vi "Norm graph.vi"(8 "error in (no error)":errorcluster, 9 "#kinetics":i32=2 min=2 step=1, 10 "Combo Box":string(combo)="Kinetics", 11 "Control-Client in":refnum<class "Control-Client.lvclass">) -> (0 "error out":errorcluster, 3 "Control-Client out":refnum<class "Control-Client.lvclass">)   [LabVIEW 2018, in "Control-Client.lvclass"]
uses:
  Control-Client.lvclass
  Control-Client.lvclass/Control-Client.ctl
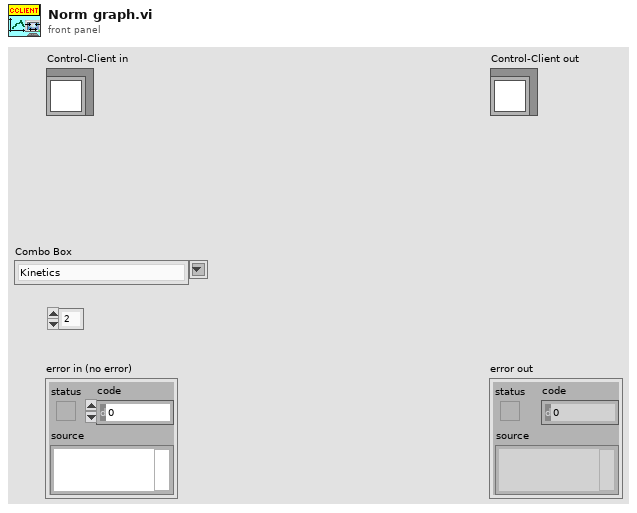
[diagram p1: front panel]
types:
  T1 = cluster{"waves slider":refnum<vi>, "times slider":refnum<vi>}
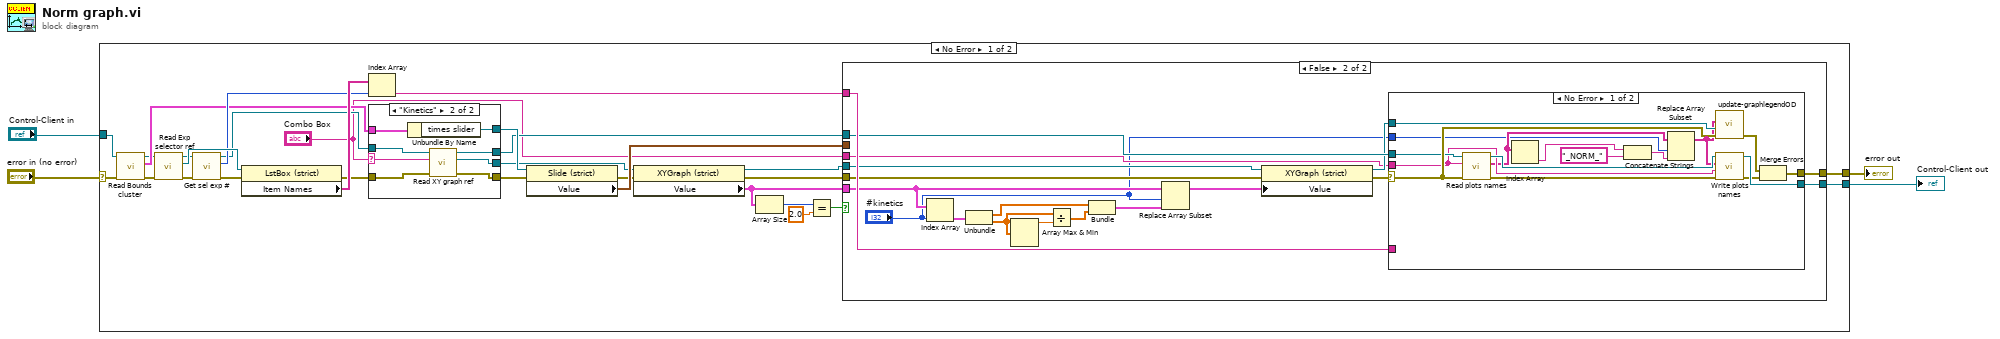
[diagram p0: block diagram]
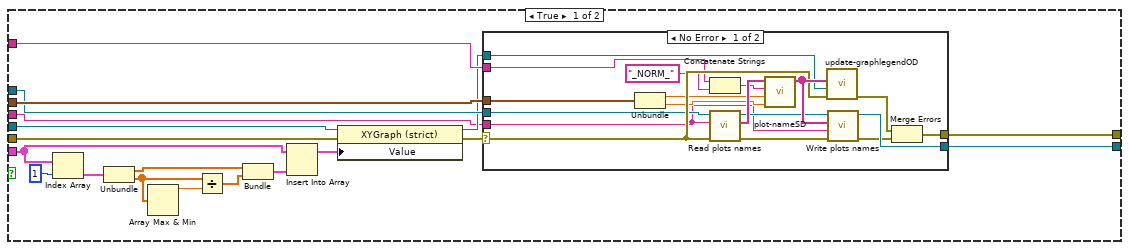
[diagram p2: hidden frame]
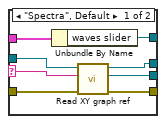
[diagram p5: hidden frame]
diagram:
  n1 = case shown="No Error" "error in (no error)" {
    selector: "error in (no error)" -> [w8 w126]
    tunnel: "Control-Client in" -> [w18 w125]
    tunnel: [w17 w126] -> w3
    tunnel: [w16 w125] -> w2
    frame No Error {
      n2 = call "Read Bounds cluster.vi"("error in (no error)"=w8, "Control-Client in"=w18) -> ("error out"=w7:errorcluster, "Bounds cluster"=w26:T1, "Control-Client out"=w9:refnum<class "Control-Client.lvclass">)  [unwired: 7 in]
      n3 = call "Read Exp selector ref.vi"("error in (no error)"=w7, "Control-Client in"=w9) -> ("error out"=w6:errorcluster, "Exp selector ref"=w30:refnum<vi>, "Control-Client out"=w10:refnum<class "Control-Client.lvclass">)  [unwired: 7 in]
      n4 = call "Get sel exp #.vi"("error in (no error)"=w6, "Control-Client in"=w10) -> ("error out"=w5:errorcluster, "Exp sel #"=w28:i32, "Control-Client out"=w24:refnum<class "Control-Client.lvclass">)  [unwired: 7 in]
      n5 = property class="LstBox (strict)"(reference=w30, error in=w5) -> (error out=w25:errorcluster, "Item Names"=w29:string[])  [unwired: 1 out]
      n6 = Index Array(array=w29, index=w28) -> (element=w31:string)
      n7 = case shown="\"Kinetics\"" "Combo Box" {
        selector: "Combo Box" -> [w116 w118]
        tunnel: [w113 w124] -> w22
        tunnel: [w112 w123] -> w27
        tunnel: w24 -> [w114 w122]
        tunnel: w25 -> [w115 w121]
        tunnel: w26 -> [w111 w120]
        tunnel: [w110 w119] -> w33
        tunnel: [w109 w117] -> w23
        frame "Spectra", Default {
          n8 = Unbundle By Name(w111) -> ("waves slider"=w110:refnum<vi>)
          n9 = call "Read XY graph ref.vi"("error in (no error)"=w115, "Combo Box"=w116, "Control-Client in"=w114) -> ("error out"=w112:errorcluster, "XY graph ref"=w113:refnum<vi>, "Control-Client out"=w109:refnum<class "Control-Client.lvclass">)  [unwired: 6 in]
        }
        frame "Kinetics" {
          n10 = Unbundle By Name(w120) -> ("times slider"=w119:refnum<vi>)
          n11 = call "Read XY graph ref.vi"("error in (no error)"=w121, "Combo Box"=w118, "Control-Client in"=w122) -> ("error out"=w123:errorcluster, "XY graph ref"=w124:refnum<vi>, "Control-Client out"=w117:refnum<class "Control-Client.lvclass">)  [unwired: 6 in]
        }
      }
      n12 = property class="Slide (strict)"(reference=w33, error in=w27) -> (error out=w20:errorcluster, "Value"=w32:cluster{dbl, dbl})  [unwired: 1 out]
      n13 = property class="XYGraph (strict)"(reference=w22, error in=w20) -> (reference out=w21:refnum<vi>, error out=w19:errorcluster, "Value"=w14:cluster{"Y":dbl[], "Y":dbl[]}[])
      n14 = Array Size(array=w14) -> (size(s)=w13:i32)
      n15 = Equal?(x=w13, y=2.0) -> (x = y?=w12:bool)
      n16 = case shown="False" w12 {
        tunnel: w32 -> [w52 _]
        tunnel: w31 -> [w51 w90]
        tunnel: w23 -> [w50 w89]
        tunnel: w21 -> [w49 w88]
        tunnel: w14 -> [w46 w77]
        tunnel: w19 -> [w44 w86]
        tunnel: [w37 w80] -> w17
        tunnel: [w36 w79] -> w16
        tunnel: "Combo Box" -> [w34 w74]
        frame True {
          n17 = Index Array(array=w46, index=1) -> (element=w42:cluster{"Y":dbl[], "Y":dbl[]})
          n18 = Unbundle(w42) -> ("Y"=w39:dbl[], "Y"=w41:dbl[])
          n19 = Array Max & Min(array=w41) -> (max value=w35:dbl)  [unwired: 3 out]
          n20 = Divide(x=w41, y=w35) -> (x/y=w40:dbl[])
          n21 = Bundle("Y"=w39, w40) -> (w38:cluster{"Y":dbl[], dbl[]})  [unwired: 1 in]
          n22 = Insert Into Array(array=w46, new element=w38) -> (w45:cluster{"Y":dbl[], "Y":dbl[]}[])  [unwired: 1 in]
          n23 = property class="XYGraph (strict)"(reference=w49, error in=w44, "Value"=w45) -> (reference out=w48:refnum<vi>, error out=w43:errorcluster)
          n24 = case shown="No Error" w43 {
            selector: w43 -> [w65 w72]
            tunnel: [w63 w72] -> w37
            tunnel: [w70 w71] -> w36
            tunnel: w52 -> [w62 _]
            tunnel: w51 -> [w59 _]
            tunnel: w50 -> [w56 w71]
            tunnel: w48 -> [w54 _]
            tunnel: w34 -> [w53 _]
            frame No Error {
              n25 = Unbundle(w62) -> (w61:dbl, w60:dbl)
              n26 = Concatenate Strings(w59, "_NORM_" ("string")) -> (w57:string)
              n27 = call "Read plots names.vi"("error in (no error)"=w65, "Combo Box"=w53, "Control-Client in"=w56) -> ("error out"=w69:errorcluster, "Plots names"=w68:string[], "Control-Client out"=w55:refnum<class "Control-Client.lvclass">)  [unwired: 6 in]
              n28 = call "plot-nameSD.vi"("To"=w60, "from"=w61, "Item name"=w57, "plot names in"=w68) -> ("plot names out"=w67:string[])  [unwired: 7 in]
              n29 = call "update-graphlegendOD.vi"("error in (no error)"=w65, "XYGraph in"=w54, "plot names"=w67) -> ("error out"=w64:errorcluster)  [unwired: 7 in]
              n30 = call "Write plots names.vi"("error in (no error)"=w69, "Combo Box"=w53, "Plot names"=w67, "Control-Client in"=w55) -> ("error out"=w66:errorcluster, "Control-Client out"=w70:refnum<class "Control-Client.lvclass">)  [unwired: 6 in]
              n31 = Merge Errors(w64, w66) -> (w63:errorcluster)
            }
            frame Error {
            }
          }
        }
        frame False {
          n32 = Index Array(array=w77, index="#kinetics") -> (element=w84:cluster{"Y":dbl[], "Y":dbl[]})
          n33 = Unbundle(w84) -> ("Y"=w81:dbl[], "Y"=w83:dbl[])
          n34 = Array Max & Min(array=w83) -> (max value=w78:dbl)  [unwired: 3 out]
          n35 = Divide(x=w83, y=w78) -> (x/y=w82:dbl[])
          n36 = Bundle("Y"=w81, w82) -> (w75:cluster{"Y":dbl[], dbl[]})  [unwired: 1 in]
          n37 = Replace Array Subset(array=w77, new element=w75, index="#kinetics") -> (w76:cluster{"Y":dbl[], "Y":dbl[]}[])
          n38 = property class="XYGraph (strict)"(reference=w88, error in=w86, "Value"=w76) -> (reference out=w87:refnum<vi>, error out=w85:errorcluster)
          n39 = case shown="No Error" w85 {
            selector: w85 -> [w103 w108]
            tunnel: [w101 w108] -> w80
            tunnel: [w106 w107] -> w79
            tunnel: w90 -> [_ _]
            tunnel: w89 -> [w99 w107]
            tunnel: w87 -> [w97 _]
            tunnel: w74 -> [w96 _]
            tunnel: "#kinetics" -> [w94 _]
            frame No Error {
              n40 = call "Read plots names.vi"("error in (no error)"=w103, "Combo Box"=w96, "Control-Client in"=w99) -> ("error out"=w105:errorcluster, "Plots names"=w95:string[], "Control-Client out"=w98:refnum<class "Control-Client.lvclass">)  [unwired: 6 in]
              n41 = Index Array(array=w95) -> (element=w93:string)  [unwired: 1 in]
              n42 = Concatenate Strings(w93, "_NORM_" ("string")) -> (w92:string)
              n43 = Replace Array Subset(array=w95, new element=w92, index=w94) -> (w91:string[])
              n44 = call "update-graphlegendOD.vi"("error in (no error)"=w103, "XYGraph in"=w97, "plot names"=w91) -> ("error out"=w102:errorcluster)  [unwired: 7 in]
              n45 = call "Write plots names.vi"("error in (no error)"=w105, "Combo Box"=w96, "Plot names"=w91, "Control-Client in"=w98) -> ("error out"=w104:errorcluster, "Control-Client out"=w106:refnum<class "Control-Client.lvclass">)  [unwired: 6 in]
              n46 = Merge Errors(w102, w104) -> (w101:errorcluster)
            }
            frame Error {
            }
          }
        }
      }
    }
    frame Error {
    }
  }
  "error out" <- w3
  "Control-Client out" <- w2
